vi "Zpos to V.vi"(3 "Z (um)":dbl=50.0) -> (0 "V":dbl=1.766)   [LabVIEW 2018]
panel:
  in  "Calibration method":u16(ring)=3 items=["Theoretical", "Experimental", "Double calibration", "Craig"]
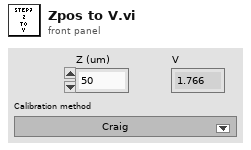
[diagram p1: front panel]
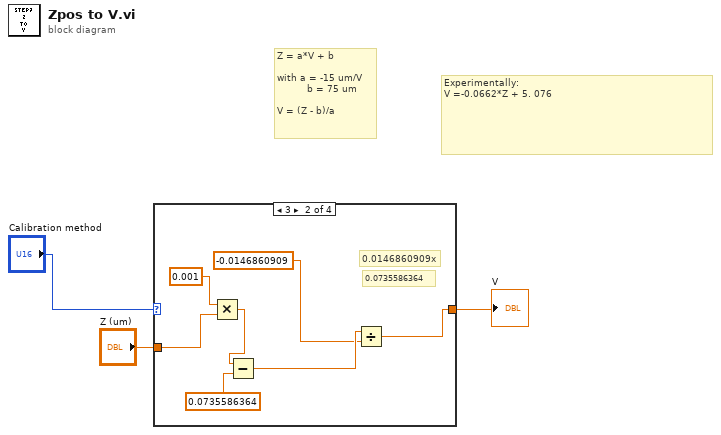
[diagram p0: block diagram]
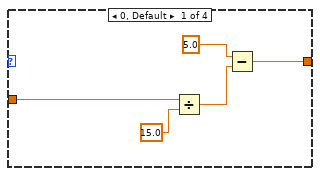
[diagram p2: hidden frame]
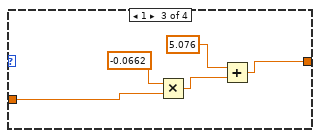
[diagram p3: hidden frame]
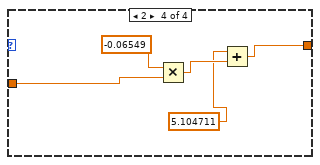
[diagram p4: hidden frame]
diagram:
  # "Experimentally:\nV =-0.0662*Z + 5. 076"
  # "Z = a*V + b\n\nwith a = -15 um/V\n          b = 75 um\n\nV = (Z - b)/a"
  n1 = case shown="3" "Calibration method" {
    tunnel: "Z (um)" -> [w8 w11 w20 w25]
    tunnel: [w6 w12 w17 w22] -> w2
    frame 0, Default {
      n2 = Divide(x=w8, y=15.0) -> (x/y=w4:dbl)
      n3 = Subtract(x=5.0, y=w4) -> (x-y=w6:dbl)
    }
    frame 3 {
      # "0.0735586364"
      # "0.0146860909x"
      n4 = Multiply(x=0.001, y=w11) -> (x*y=w9:dbl)
      n5 = Subtract(x=w9, y=0.0735586364) -> (x-y=w14:dbl)
      n6 = Divide(x=w14, y=-0.0146860909) -> (x/y=w12:dbl)
    }
    frame 1 {
      n7 = Multiply(x=-0.0662, y=w20) -> (x*y=w18:dbl)
      n8 = Add(x=5.076, y=w18) -> (x+y=w17:dbl)
    }
    frame 2 {
      n9 = Multiply(x=-0.06549, y=w25) -> (x*y=w23:dbl)
      n10 = Add(x=5.104711, y=w23) -> (x+y=w22:dbl)
    }
  }
  "V" <- w2
